vi "Send speed logging start notifier in live protocols.vi"   [LabVIEW 2017]
uses:
  Typedefs/Speed acq notifier data.ctl
  Typedefs/Notifier Function.ctl
types:
  T1 = typedef "Notifier Function.ctl" = enum16{"Send notifier", "Wait on notification", "Release notifier"}
  T2 = typedef "Speed acq notifier data.ctl" = cluster{"Log speed data":bool, "File path":path, "Initial timestamp":timestamp}
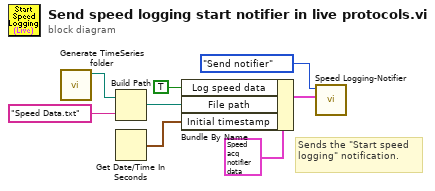
[diagram p0: block diagram]
diagram:
  # "Sends the \"Start speed logging\" notification."
  n1 = call "Generate TimeSeries folder.vi"() -> ("Timelapse folder path"=w5:path)  [unwired: 10 in, 1 out]
  n2 = Build Path(base path=w5, name or relative path="Speed Data.txt") -> (appended path=w7:path)
  n3 = Get Date/Time In Seconds() -> (seconds since 1Jan1904=w1:timestamp)
  n4 = Bundle By Name(cluster=T2 {"Log speed data"=FALSE, "File path"=path "", "Initial timestamp"=timestamp(0 s since 1904-01-01)} ("Value to send"), "Log speed data"=TRUE ("Log?"), "File path"=w7, "Initial timestamp"=w1) -> (w4:T2)
  n5 = call "Speed Logging-Notifier.vi"("Value to send"=w4, "Notifier Function"=Notifier_Function."Send notifier") -> ()  [unwired: 7 in, 3 out]
